vi "SELECT SQL.vi"(11 "INVENTARIO":string="INVENTARIO_1") -> (1 "PRODUCTO":string[](array[string]), 2 "MONEDA":string[](array[string]), 3 "CANTIDAD":i64[](array[numeric]), 4 "COSTO":i64[](array[numeric]))   [LabVIEW 2019]
uses:
  <vilib>/drjdpowell/SQLite Library/SQL Connection/Open (path).vi
  <vilib>/drjdpowell/SQLite Library/SQL Connection/Open (string).vi
  <vilib>/AdvancedString/Path To Command Line String.vi
  <vilib>/drjdpowell/SQLite Library/SQL Connection/Execute SQL (1D String).vi
  <vilib>/drjdpowell/SQLite Library/SQL Connection/Execute SQL (1D Integer results).vi
  <vilib>/drjdpowell/SQLite Library/SQL Connection/Connection.lvclass
  <vilib>/drjdpowell/SQLite Library/SQLite.lvlib
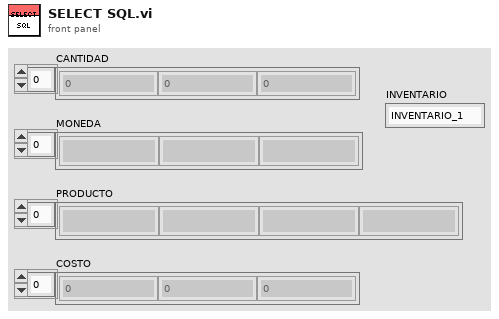
[diagram p1: front panel]
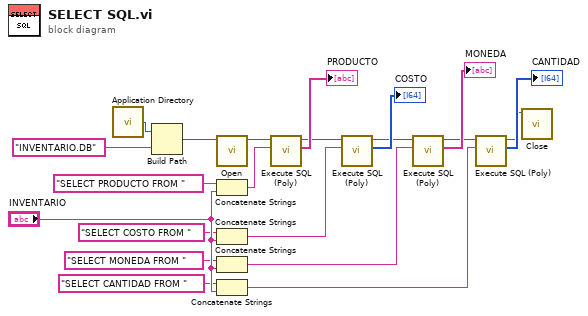
[diagram p0: block diagram]
diagram:
  n1 = call <vilib>:"Application Directory.vi"() -> ("Application Directory"=w1:path)
  n2 = Build Path(base path=w1, name or relative path="INVENTARIO.DB") -> (appended path=w2:path)
  n3 = call-poly <vilib>:"Open.vi"("db file"=w2) -> ("SQLite Connection"=w3:refnum<class "Connection.lvclass">)  [unwired: 9 in, 1 out]
  n4 = Concatenate Strings("SELECT PRODUCTO FROM " ("string"), "INVENTARIO") -> (w6:string)
  n5 = Concatenate Strings("SELECT COSTO FROM " ("string"), "INVENTARIO") -> (w14:string)
  n6 = Concatenate Strings("SELECT MONEDA FROM " ("string"), "INVENTARIO") -> (w15:string)
  n7 = Concatenate Strings("SELECT CANTIDAD FROM " ("string"), "INVENTARIO") -> (w16:string)
  n8 = call-poly <vilib>:"Execute SQL (Poly).vi"("SQL"=w6, "SQLite Connection in"=w3) -> ("Result Set"=→"PRODUCTO":string[], "SQLite Connection"=w7:refnum<class "Connection.lvclass">)  [unwired: 6 in, 2 out]
  n9 = call-poly <vilib>:"Execute SQL (Poly).vi"("SQL"=w14, "SQLite Connection in"=w7) -> ("Result Set"=→"COSTO":i64[], "SQLite Connection"=w8:refnum<class "Connection.lvclass">)  [unwired: 6 in, 2 out]
  n10 = call-poly <vilib>:"Execute SQL (Poly).vi"("SQL"=w15, "SQLite Connection in"=w8) -> ("Result Set"=→"MONEDA":string[], "SQLite Connection"=w9:refnum<class "Connection.lvclass">)  [unwired: 6 in, 2 out]
  n11 = call-poly <vilib>:"Execute SQL (Poly).vi"("SQL"=w16, "SQLite Connection in"=w9) -> ("Result Set"=→"CANTIDAD":i64[], "SQLite Connection"=w17:refnum<class "Connection.lvclass">)  [unwired: 6 in, 2 out]
  n12 = call-dynamic "Close.vi"("SQLite Connection in"=w17) -> ()  [unwired: 10 in, 1 out]
